vi "AdjustedHeading.vi"(1 "Heading In":dbl) -> (0 "Heading Out":dbl)   [LabVIEW 2012]
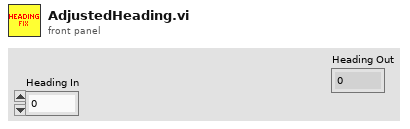
[diagram p1: front panel]
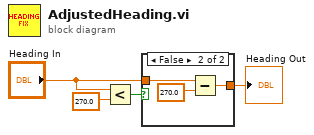
[diagram p0: block diagram]
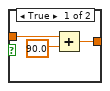
[diagram p2: hidden frame]
diagram:
  n1 = Less?(x="Heading In", y=270.0) -> (x < y?=w3:bool)
  n2 = case shown="False" w3 {
    tunnel: "Heading In" -> [w7 w10]
    tunnel: [w5 w8] -> w1
    frame True {
      n3 = Add(x=w7, y=90.0) -> (x+y=w5:dbl)
    }
    frame False {
      n4 = Subtract(x=w10, y=270.0) -> (x-y=w8:dbl)
    }
  }
  "Heading Out" <- w1
